vi "Pre-Actor.vi"(8 "error in":errorcluster, 11 "PRM in":refnum<class "PRM.lvclass">) -> (0 "error out":errorcluster, 3 "PRM out":refnum<class "PRM.lvclass">)   [LabVIEW 2019, in "PRM.lvlib" / "PRM.lvclass"]
doc: "This override VI is to provide the means for children classes to perform application specific post launch initialization functions that must be performed *prior* to calling the actor. \n\n***DO NOT USE THE CHECK FOR FAULT ROUTINE HERE***"
uses:
  Library/PRM.lvclass
  builds/Instruments/Instruments.lvlibp/Library/Instruments.lvclass
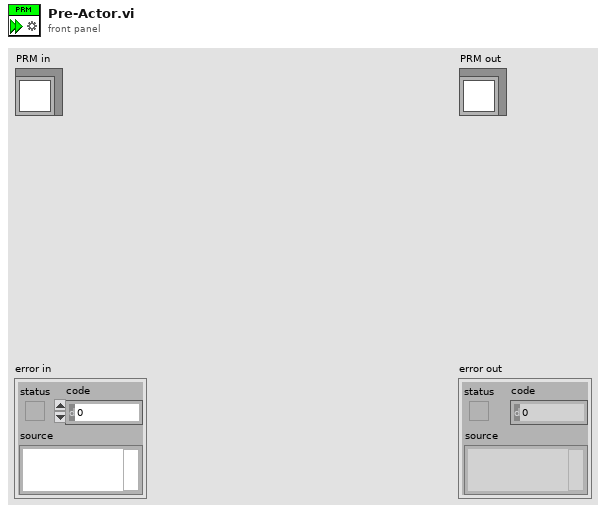
[diagram p1: front panel]
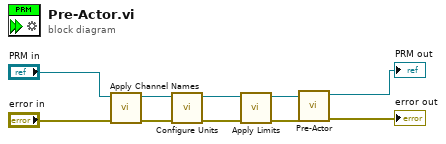
[diagram p0: block diagram]
diagram:
  n1 = call "Apply Channel Names.vi"("error in"="error in", "PRM in"="PRM in") -> ("error out"=w5:errorcluster, "PRM out"=w6:refnum<class "PRM.lvclass">)  [unwired: 8 in]
  n2 = call "Configure Units.vi"("error in"=w5, "PRM in"=w6) -> ("error out"=w3:errorcluster, "PRM out"=w4:refnum<class "PRM.lvclass">)  [unwired: 8 in]
  n3 = call "Apply Limits.vi"("error in"=w3, "PRM in"=w4) -> ("error out"=w1:errorcluster, "PRM out"=w2:refnum<class "PRM.lvclass">)  [unwired: 8 in]
  n4 = call-parent "Pre-Actor.vi"("error in (no error)"=w1, "Instruments in"=w2) -> ("error out"=→"error out":errorcluster, "Instruments out"=→"PRM out":refnum<class "PRM.lvclass">)  [unwired: 8 in]
